vi "Add Node and Return ID.vi"(11 "Abstract Graph in":refnum<class "Abstract Graph.lvclass">) -> (1 "Node Already Existed":bool, 2 "Node ID":string, 3 "Abstract Graph out":refnum<class "Abstract Graph.lvclass">)   [LabVIEW 2021, in "GraphLib.lvlib" / "Abstract Graph.lvclass"]
uses:
  Abstract Graph.lvclass
  Node.ctl
  GraphLib.lvlib
panel:
  out "Node":T1
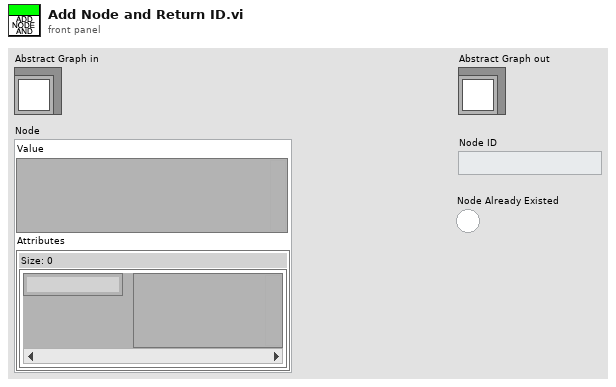
[diagram p1: front panel]
types:
  T1 = typedef "GraphLib.lvlib/Node.ctl" = cluster{"Value":variant, "Attributes":map{string, variant}}
  T2 = typedef "GraphLib.lvlib/Node Internal.ctl" = cluster{"Node":T1, "Edge IDs":set{string}}
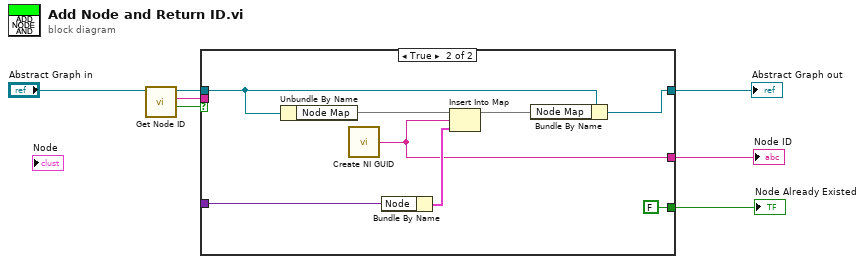
[diagram p0: block diagram]
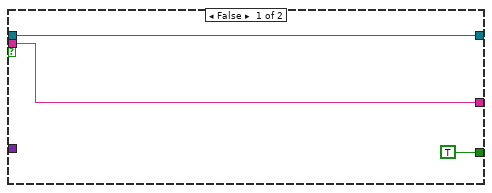
[diagram p2: hidden frame]
diagram:
  n1 = call "Get Node ID.vi"("Abstract Graph in"="Abstract Graph in") -> ("Node Exist"=w7:bool, "Node ID"=w6:string, "Abstract Graph out"=w5:refnum<class "Abstract Graph.lvclass">)  [unwired: 8 in]
  n2 = case shown="True" w7 {
    tunnel: w6 -> [w10 _]
    tunnel: w5 -> [w11 w16]
    tunnel: [_ w18] -> w4
    tunnel: [w11 w14] -> w3
    tunnel: [w10 w13] -> w2
    tunnel: [TRUE FALSE] -> w1
    frame False {
    }
    frame True {
      n3 = Unbundle By Name(w16) -> ("Node Map"=w19:map{string, T2})
      n4 = call <vilib>:"Create NI GUID.vi"() -> ("NI GUID"=w13:string)
      n5 = Bundle By Name("Node"=w18) -> (w17:cluster{})  [unwired: 1 in]
      n6 = Insert Into Map(map in=w19, key=w13, value=w17) -> (map out=w15:map{string, T2})  [unwired: 2 out]
      n7 = Bundle By Name(cluster=w16, "Node Map"=w15) -> (w14:refnum<class "Abstract Graph.lvclass">)
    }
  }
  "Abstract Graph out" <- w3
  "Node ID" <- w2
  "Node Already Existed" <- w1
